vi "initialise pretomo values.vi"(8 "error in (no error)":errorcluster, 11 "Tomo in":refnum<class "Tomo.lvclass">) -> (0 "error out":errorcluster, 3 "Tomo out":refnum<class "Tomo.lvclass">)   [LabVIEW 2012, in "Tomo.lvclass"]
uses:
  Tomo.lvclass
  Tomo.lvclass/Tomo.ctl
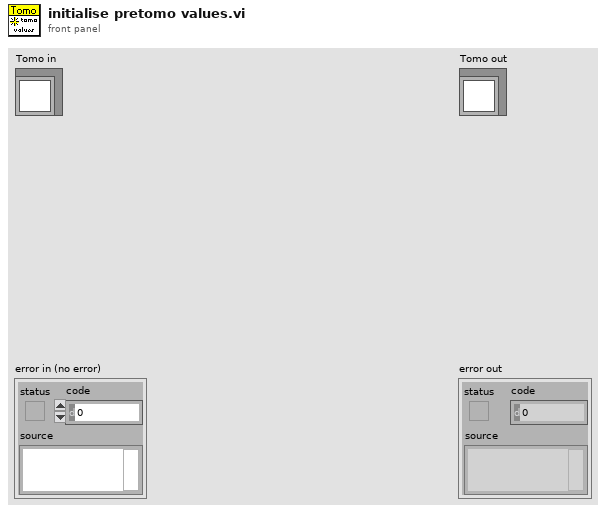
[diagram p1: front panel]
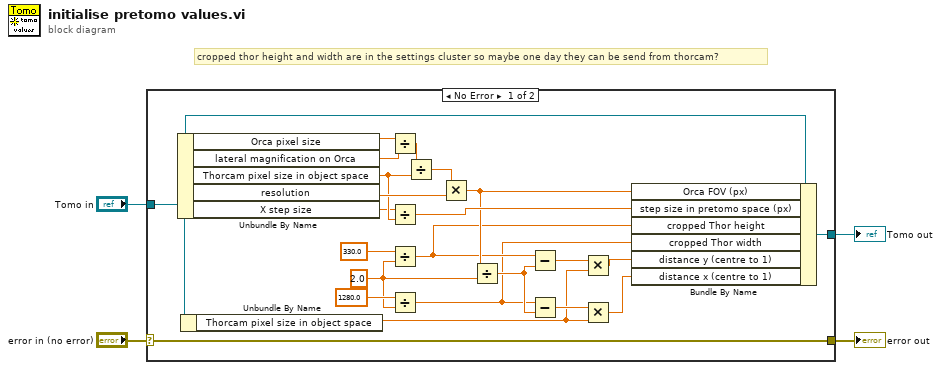
[diagram p0: block diagram]
diagram:
  # "cropped thor height and width are in the settings cluster so maybe one day they can be send from thorcam?"
  n1 = case shown="No Error" "error in (no error)" {
    selector: "error in (no error)" -> [w27 w29]
    tunnel: [w27 w29] -> w3
    tunnel: [w21 w28] -> w1
    tunnel: "Tomo in" -> [w15 w28]
    frame No Error {
      w7 = 2.0 ("y")
      n2 = Unbundle By Name(w15) -> ("Orca pixel size"=w26:dbl[unit], "lateral magnification on Orca"=w25:dbl, "Thorcam pixel size in object space"=w20:dbl[unit], "resolution"=w22:dbl, "X step size"=w12:dbl[unit])
      n3 = Unbundle By Name(w15) -> ("Thorcam pixel size in object space"=w13:dbl[unit])
      n4 = Divide(x=w26, y=w25) -> (x/y=w24:dbl[unit])
      n5 = Divide(x=w12, y=w20) -> (x/y=w19:dbl)
      n6 = Divide(x=330.0 ("settings.cropped Thor height"), y=w7) -> (x/y=w10:dbl)
      n7 = Divide(x=1280.0 ("settings.cropped Thor width"), y=w7) -> (x/y=w8:dbl)
      n8 = Divide(x=w24, y=w20) -> (x/y=w23:dbl)
      n9 = Multiply(x=w23, y=w22) -> (x*y=w14:dbl)
      n10 = Divide(x=w14, y=w7) -> (x/y=w18:dbl)
      n11 = Subtract(x=w10, y=w18) -> (x-y=w17:dbl)
      n12 = Subtract(x=w8, y=w18) -> (x-y=w16:dbl)
      n13 = Multiply(x=w17, y=w13) -> (x*y=w6:dbl[unit])
      n14 = Multiply(x=w16, y=w13) -> (x*y=w5:dbl[unit])
      n15 = Bundle By Name(cluster=w15, "Orca FOV (px)"=w14, "step size in pretomo space (px)"=w19, "cropped Thor height"=w10, "cropped Thor width"=w8, "distance y (centre to 1)"=w6, "distance x (centre to 1)"=w5) -> (w21:refnum<class "Tomo.lvclass">)
    }
    frame Error {
    }
  }
  "error out" <- w3
  "Tomo out" <- w1
